vi "Set Result Collector.vi"(8 "error in (no error)":errorcluster, 10 "Test Suite":refnum<class "Result Collector.lvclass">, 11 "Slave Test Runner In":refnum<class "Slave Test Runner.lvclass">) -> (0 "error out":errorcluster, 3 "Slave Test Runner Out":refnum<class "Slave Test Runner.lvclass">)   [LabVIEW 2020, in "Slave Test Runner.lvclass"]
uses:
  Slave Test Runner.lvclass
  Application Framework/Process Classes/Process/Process.lvclass
  Result Collector/Result Collector.lvclass
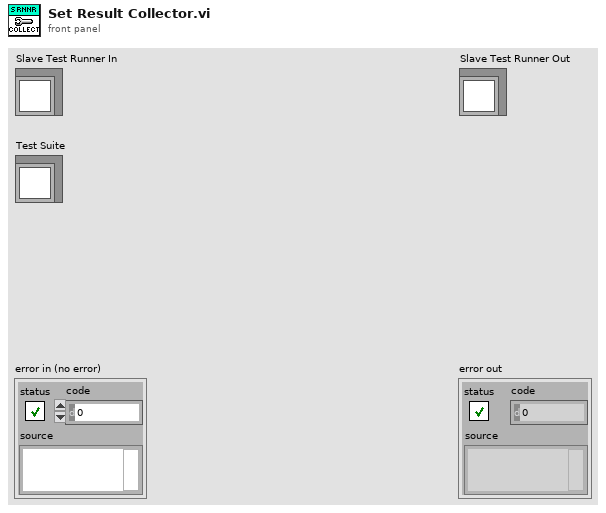
[diagram p1: front panel]
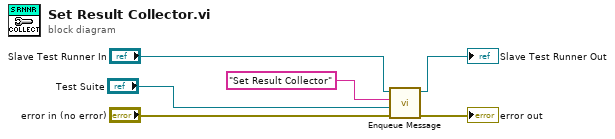
[diagram p0: block diagram]
diagram:
  n1 = call "Enqueue Message.vi"("error in (no error)"="error in (no error)", "Message Data"="Test Suite", "Message"="Set Result Collector", "Process In"="Slave Test Runner In") -> ("error out"=→"error out":errorcluster, "Process Out"=→"Slave Test Runner Out":refnum<class "Slave Test Runner.lvclass">)  [unwired: 6 in]
